vi "File New.vi"(0 "VISA resource name":refnum<visa-resource-name>, 5 "File Number (1)":i32=1, 7 "File Name":string, 11 "error in (no error)":errorcluster) -> (4 "VISA resource name out":refnum<visa-resource-name>, 15 "error out":errorcluster)   [LabVIEW 2020, in "Associated Research 78XX Series.lvlib"]
doc: "FN {<file number>,<file name>}\nCreates a new file name at the specified file number.s\n\nIf there is a file already located at the desired number it will be moved to the next higher number and inserted in its place. New files can be added to the bottom of the file list but there must not be any numbers that do not have a file defined."
uses:
  <instrlib>/Associated Research 78XX Series/Associated Research 78XX Series.lvlib
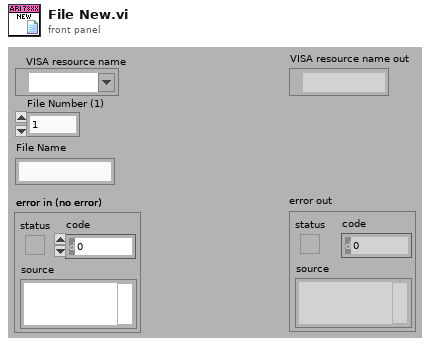
[diagram p1: front panel]
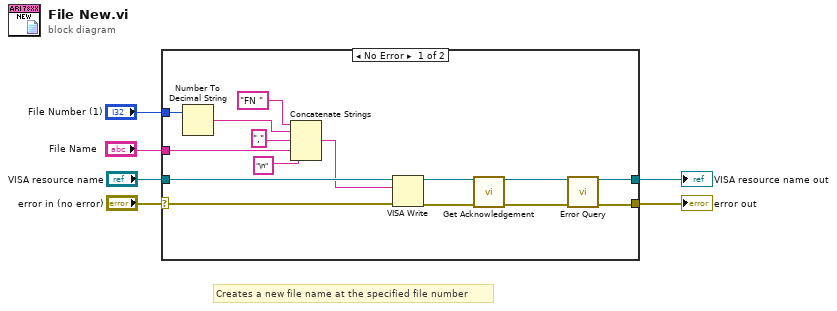
[diagram p0: block diagram]
diagram:
  # "Creates a new file name at the specified file number"
  n1 = case shown="No Error" "error in (no error)" {
    selector: "error in (no error)" -> [w18 w23]
    tunnel: [w19 w23] -> w5
    tunnel: [w20 w22] -> w3
    tunnel: "VISA resource name" -> [w21 w22]
    tunnel: "File Name" -> [w12 _]
    tunnel: "File Number (1)" -> [w11 _]
    frame No Error {
      n2 = Number To Decimal String(number=w11) -> (decimal integer string=w15:string)  [unwired: 1 in]
      n3 = Concatenate Strings("FN " ("\"False\" Command"), w15, "," ("Substring"), w12, "\n" ("string")) -> (w13:string)
      n4 = VISA Write(VISA resource name=w21, write buffer=w13, error in (no error)=w18) -> (VISA resource name out=w8:refnum<visa-resource-name>, error out=w7:errorcluster)  [unwired: 1 out]
      n5 = call <instrlib>:"Get Acknowledgement.vi"("VISA resource name"=w8, "error in (no error)"=w7) -> ("VISA resource name out"=w10:refnum<visa-resource-name>, "error out"=w9:errorcluster)  [unwired: 12 in]
      n6 = call <instrlib>:"Error Query.vi"("VISA resource name"=w10, "error in (no error)"=w9) -> ("VISA resource name out"=w20:refnum<visa-resource-name>, "error out"=w19:errorcluster)  [unwired: 10 in, 2 out]
    }
    frame Error {
    }
  }
  "error out" <- w5
  "VISA resource name out" <- w3
